vi "Pre Launch Init.vi"(11 "CS++Motor in":refnum<class "CS++Motor.lvclass">) -> (0 "error out":errorcluster, 3 "CS++Motor out":refnum<class "CS++Motor.lvclass">)   [LabVIEW 2015, in "CS++Motor.lvlib" / "CS++Motor.lvclass"]
doc: "(<B>Filename</B>: Actor Framework.lvlib:Actor.lvclass:Pre Launch Init.vi)\n\nDefines behavior that occurs after the Launch Actor method is invoked but before the actor's Actor Core method begins running.\n\nThe Pre Launch Init method is guaranteed to finish before the Launch Actor method returns to its caller and before the actor itself receives any messages. Any references that the Pre Launch Init method obtains are guaranteed to have the same lifetime as the actor itself. Any errors that the Pre Launch Init method returns will abort the launch.\n\nBy default, this method does nothing. A descendant class may override it to define behavior."
uses:
  CS++Motor.lvclass
  CS++Motor.lvclass/CS++Motor.ctl
  CSPP_Core/Actors/CS++DeviceActor/CS++DeviceActor.lvclass
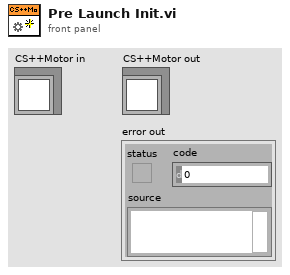
[diagram p1: front panel]
types:
  T1 = cluster{"Command":string, "AxisNumber":u8, "Data":variant}
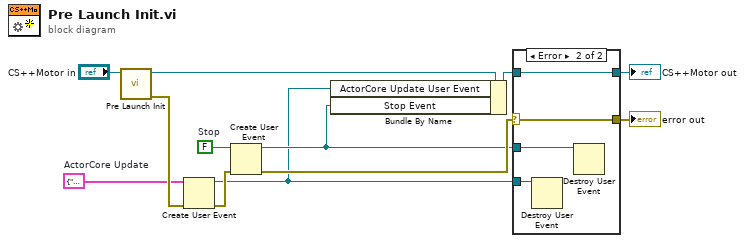
[diagram p0: block diagram]
diagram:
  w1 = T1 {"Command"="", "AxisNumber"=0, "Data"=variant}  # ActorCore Update
  w9 = FALSE  # Stop
  n1 = call-parent "Pre Launch Init.vi"("CS++BaseActor in"="CS++Motor in") -> ("error out"=w8:errorcluster, "CS++BaseActor out"=w12:refnum<class "CS++Motor.lvclass">)  [unwired: 9 in]
  n2 = Create User Event(user event datatype=w1, error in=w8) -> (user event=w2:refnum<user-event>, error out=w10:errorcluster)
  n3 = Create User Event(user event datatype=w9, error in=w10) -> (user event=w3:refnum<user-event>, error out=w4:errorcluster)
  n4 = Bundle By Name(cluster=w12, "ActorCore Update User Event"=w2, "Stop Event"=w3) -> (w7:refnum<class "CS++Motor.lvclass">)
  n5 = case shown="Error" w4 {
    selector: w4 -> [w14 w17]
    tunnel: [w14 w17] -> w5
    tunnel: [w13 w18] -> w6
    tunnel: w7 -> [w13 w18]
    tunnel: w3 -> [_ w16]
    tunnel: w2 -> [_ w15]
    frame No Error {
    }
    frame Error {
      n6 = Destroy User Event(user event=w15) -> ()  [unwired: 1 in, 1 out]
      n7 = Destroy User Event(user event=w16) -> ()  [unwired: 1 in, 1 out]
    }
  }
  "error out" <- w5
  "CS++Motor out" <- w6
